vi "LinearFilter_LowPassBW1.vi"(9 "SamplePeriod":dbl format="%13.5p", 11 "TimeConstant":dbl format="%13.5p") -> (3 "LINEAR_FILTER":T1 {"Outputs" format="%13.5g"; "Inputs" format="%13.5g"; "OutputGains" format="%13.5g"; "InputGains" format="%13.5g"})   [LabVIEW 2023]
doc: "Creates a 1st order Butterworth low pass filter.\n\nMore information on this type of filter can be found at:\n\n https://en.wikipedia.org/wiki/Butterworth_filter\n\nInputs: \n - timeConstant - The discrete-time time constant in seconds.\n -samplePeriod - The period in seconds between samples taken by the user.\n\nOutputs:\n - LinearFilter - Created datat structure"
uses:
  <vilib>/Rock Robotics/WPI/ThirdParty/JAS_Junk/TrajLib/TypeDef/LINEAR_FILTER.ctl
  <vilib>/Rock Robotics/SystemInterfaces/NetworkCommunication/NetComm_UsageReport_report.vi
  <vilib>/Rock Robotics/WPI/ThirdParty/JAS_Junk/TrajLib/Globals/Util_LibraryGlobals.vi
  <vilib>/Rock Robotics/WPI/ThirdParty/JAS_Junk/TrajLib/Trajectory_Library.lvlib
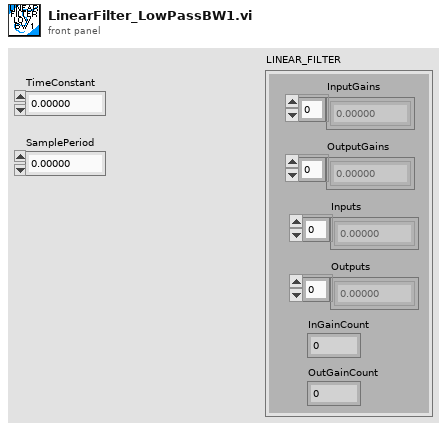
[diagram p1: front panel]
types:
  T1 = typedef "Trajectory_Library.lvlib/LINEAR_FILTER.ctl" = cluster{"InputGains":dbl[], "OutputGains":dbl[], "Inputs":dbl[], "Outputs":dbl[], "InGainCount":i32, "OutGainCount":i32}
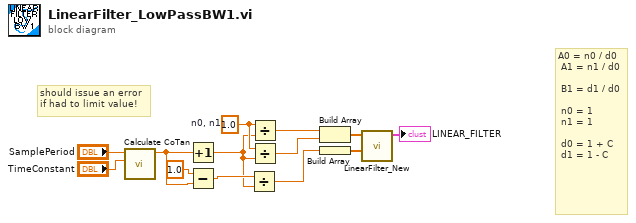
[diagram p0: block diagram]
diagram:
  w4 = 1.0  # n0, n1
  # "should issue an error\nif had to limit value!"
  # "A0 = n0 / d0\n\tA1 = n1 / d0\n\n\tB1 = d1 / d0\n\n\tn0 = 1\n\tn1 = 1\n\n\td0 = 1 + C\n\td1 = 1 - C"
  n1 = call "Calculate CoTan.vi"("TimeConstant (sec)"="TimeConstant", "SamplePeriod (sec)"="SamplePeriod") -> ("C"=w9:dbl)  [unwired: 8 in, 1 out]
  n2 = Increment(x=w9) -> (x+1=w3:dbl)
  n3 = Subtract(x=1.0, y=w9) -> (x-y=w5:dbl)
  n4 = Divide(x=w5, y=w3) -> (x/y=w8:dbl)
  n5 = Divide(x=w4, y=w3) -> (x/y=w2:dbl)
  n6 = Divide(x=w4, y=w3) -> (x/y=w1:dbl)
  n7 = Build Array(w2, w1) -> (w13:dbl[])
  n8 = Build Array(w8) -> (w11:dbl[])
  n9 = call <vilib>:"LinearFilter_New.vi"("OutputGains"=w11, "InputGains"=w13) -> ("LINEAR_FILTER"=→"LINEAR_FILTER":T1)  [unwired: 9 in]
